vi "Periodic Tasks.vi"(8 "error in":errorcluster) -> ()   [LabVIEW 2018]
doc: "This VI runs in parallel to other tasks. It can contain as many user-defined periodic loops as you need. These can carry out PID or other sorts of timed response."
uses:
  <vilib>/Rock Robotics/WPI/ThirdParty/Phoenix-LabVIEW/Motor Controller/Controls/CTRE_Phoenix_MotorControl_ControlMode.ctl
  Robot Global Data.vi
  <vilib>/addons/control/pid/pid.llb/PID (DBL).vi
  <vilib>/Rock Robotics/WPI/ThirdParty/Phoenix-LabVIEW/Motor Controller/Get/CTRE_Phoenix_MotorController_GetVoltage.vi
  <vilib>/addons/control/pid/NI_PID_pid.lvlib
  <vilib>/Rock Robotics/SystemInterfaces/DIO/FPGA_DIOChannel.ctl
panel:
  in  "Front Center":i16=-81
  in  "Rear Center":i16=256
  out "Rear Encoder":i16=8
  out "Rear Encoder":dbl(graph)=8.0
  out "Front Encoder":i16=8
  out "Front Encoder":dbl(graph)=8.0
  in  "Initial Count":i32
  out "Count":dbl=-1091.0
  out "PID Output 2":dbl(graph)=0.5
  in  "Hue":cluster{dbl, dbl}(slide)={0.0, 5.05050505050505} scale=0.0..10.0
  in  "Saturation":cluster{dbl, dbl}(slide)={0.0, 5.05050505050505} scale=0.0..10.0
  in  "Value":cluster{dbl, dbl}(slide)={0.0, 5.05050505050505} scale=0.0..10.0
  in  "Count Offset":i32
  out "Counts":i32=1466
  out "Count State":dbl=-1091.0
  in  "Bucket PID":T1={"proportional gain (Kc)"=0.7, "integral time (Ti, min)"=0.0, "derivative time (Td, min)"=0.0}
  in  "PID Range":cluster{"output high":dbl, "output low":dbl}={"output high"=0.7, "output low"=-0.7} {"output low" format="%.2f"; "output high" format="%.2f"}
  out "PID Output":dbl(graph)=0.5
  out "PID Inputs":cluster{dbl, "Bucket Angle ":dbl}(graph)={-2182.0, "Bucket Angle "=0.0}
  out "Count Chart":cluster{dbl, "Value":i32}(graph)
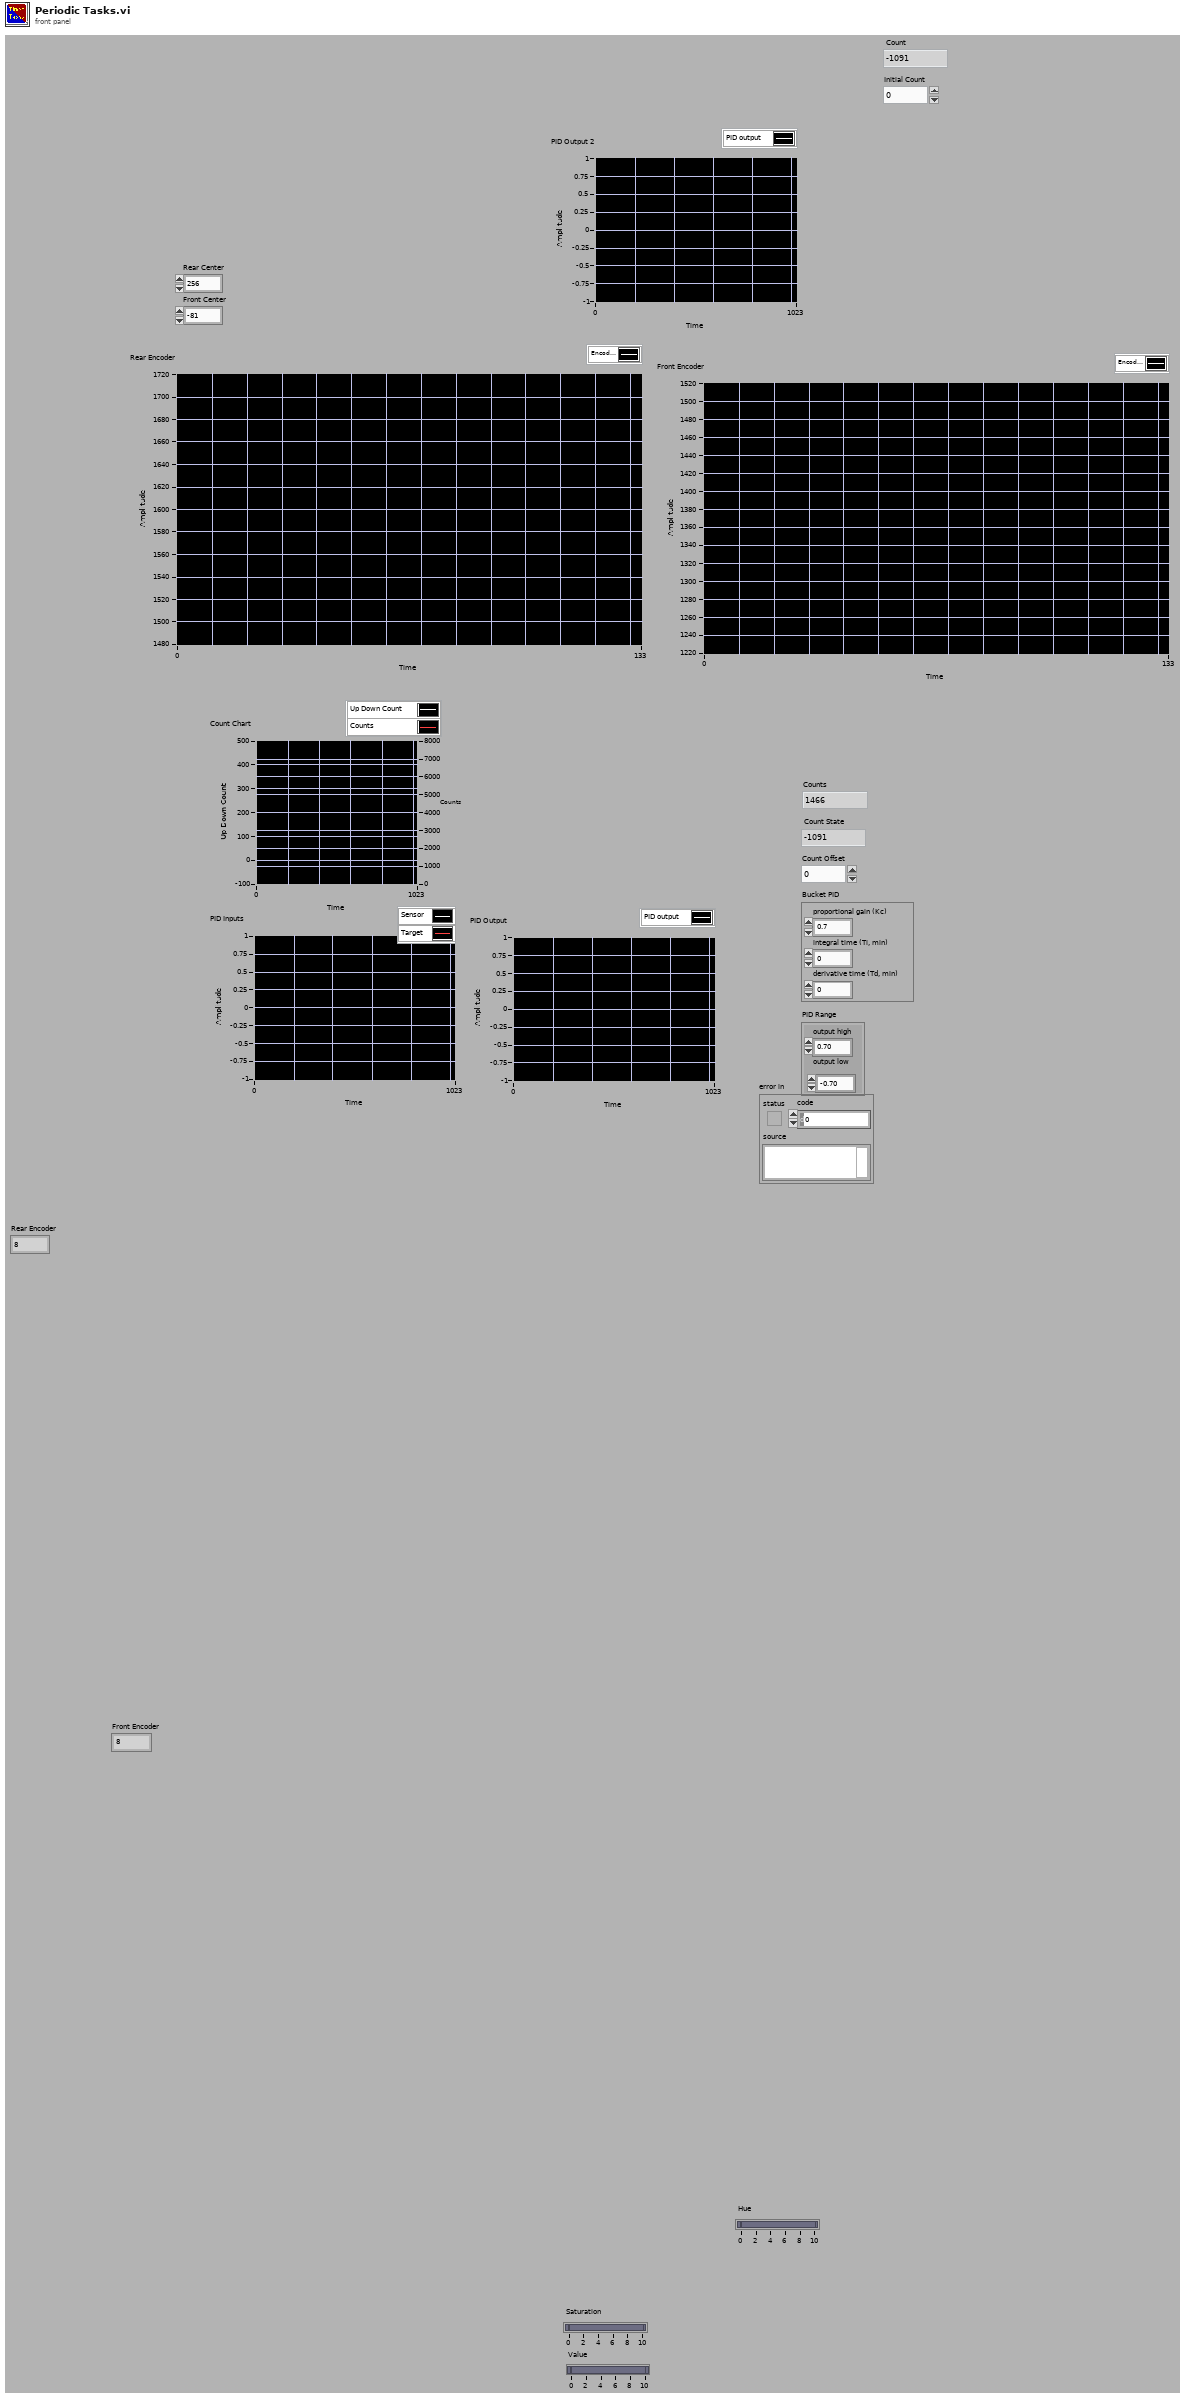
[diagram p1: front panel]
types:
  T1 = cluster{"proportional gain (Kc)":dbl, "integral time (Ti, min)":dbl, "derivative time (Td, min)":dbl}
  T2 = typedef "WPI_EncoderDevRef.ctl" = cluster{"DevStatus":errorcluster, "EncoderIndex":T3, "CounterIndex":T4, "DistancePerCount":dbl, "Decoding Type":T5}
  T3 = typedef "FPGA_EncoderIdx.ctl" = enum8{"Enc 0", "Enc 1", "Enc 2", "Enc 3", "Enc 4", "Enc 5", "Enc 6", "Enc 7", "Invalid"}
  T4 = typedef "FPGA_CounterCtrSystemIndex.ctl" = enum8{"Ctr 0", "Ctr 1", "Ctr 2", "Ctr 3", "Ctr 4", "Ctr 5", "Ctr 6", "Ctr 7", "Invalid"}
  T5 = typedef "WPI_EncoderType.ctl" = enum16{"1x", "2x", "4x"}
  T6 = typedef "WPI_MotorControlDeviceRef.ctl" = cluster{"DeviceStatus":errorcluster, "Type":T7, "PWM":cluster{"PWM Channel":T8, "DeadBand":T9}, "CAN":cluster{"Device Number":u8, "SetOutput VI Ref":variant, "GetOutput VI Ref":variant, "Enable VI Ref":variant, "Disable VI Ref":variant, "Data":variant}, "Invert":bool, "DIO PWM":cluster{"PWM \"Enable\" Channel":T8, "DIOChannel":T10, "PWM Rate":dbl}}
  T7 = typedef "WPI_MotorControlType.ctl" = enum16{"PWM", "CAN", "DIO PWM"}
  T8 = typedef "FPGA_DIOPWMChannel.ctl" = enum8{"PWM 0", "PWM 1", "PWM 2", "PWM 3", "PWM 4", "PWM 5", "PWM 6", "PWM 7", "PWM 8", "PWM 9", "PWM MXP 0", "PWM MXP 1", "PWM MXP 2", "PWM MXP 3", "PWM MXP 4", "PWM MXP 5", "PWM MXP 6", "PWM MXP 7", "PWM MXP 8", "PWM MXP 9", "Invalid"}
  T9 = typedef "WPI_PWMDeadband.ctl" = cluster{"Name":string, "maxPositivePwm":i32, "minPositivePwm":i32, "centerPwm":i32, "maxNegativePwm":i32, "minNegativePwm":i32, "angularRange":u16}
  T10 = typedef "FPGA_DIOChannel.ctl" = enum8{"DIO 0", "DIO 1", "DIO 2", "DIO 3", "DIO 4", "DIO 5", "DIO 6", "DIO 7", "DIO 8", "DIO 9", "DIO MXP 0", "DIO MXP 1", "DIO MXP 2", "DIO MXP 3", "DIO MXP 4", "DIO MXP 5", "DIO MXP 6", "DIO MXP 7", "DIO MXP 8", "DIO MXP 9", "DIO MXP 10", "DIO MXP 11", "DIO MXP 12", "DIO MXP 13", "DIO MXP 14", "DIO MXP 15", "SPI Port CS1", "SPI Port CS2", "SPI Port CS3", "SPI Port MISO", "SPI Port MOSI", "Invalid"}
  T11 = typedef "WPI_CounterDevRef.ctl" = cluster{"DevStatus":errorcluster, "CntIndex":T4}
  T12 = typedef "WPI_DigitalOutputDevRef.ctl" = cluster{"DIO Channel":T10, "DevStatus":errorcluster}
  T13 = typedef "CTRE_Phoenix_MotorControl_ControlMode.ctl" = u16
  T14 = typedef "WPI_SwitchDevRef.ctl" = cluster{"DevStatus":errorcluster, "DIO Channel":T10, "CntIndex":T4, "Normally Closed":bool}
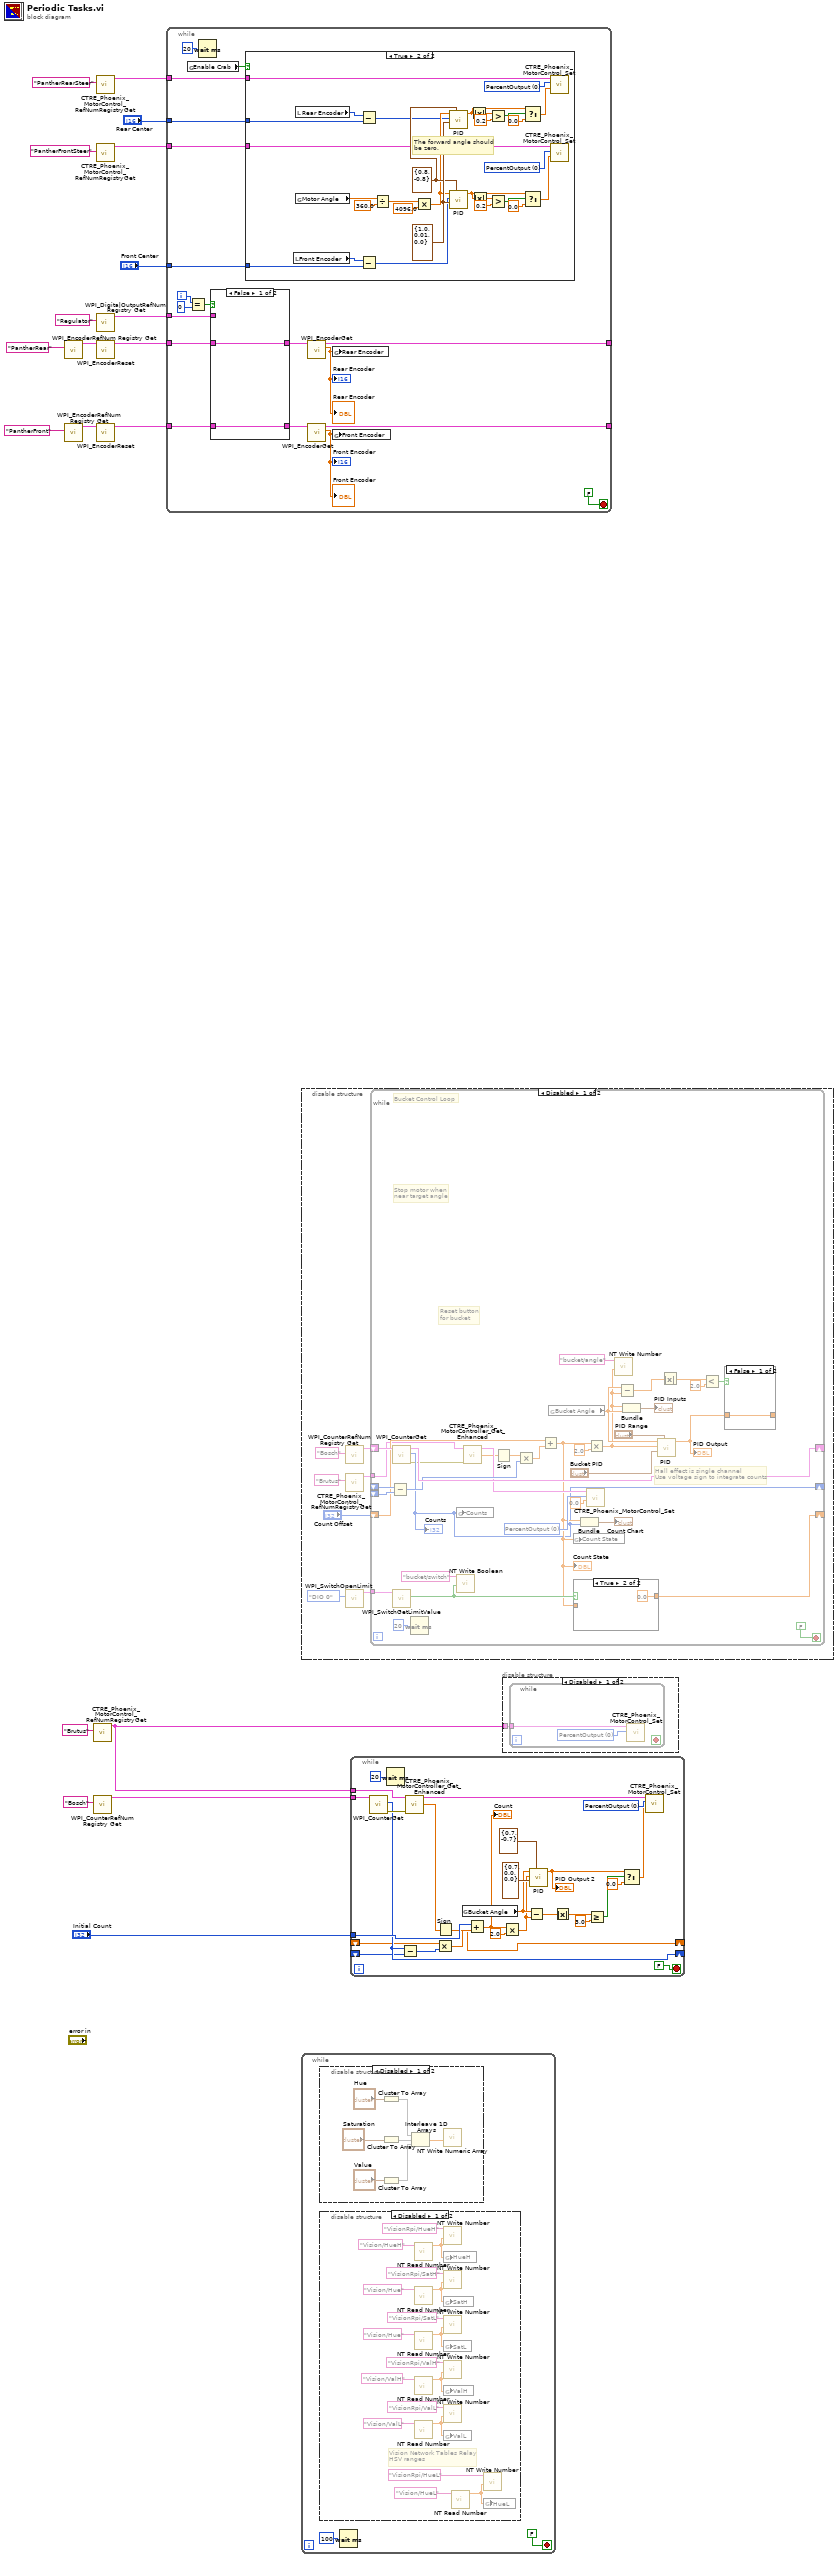
[diagram p0: block diagram]
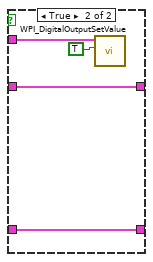
[diagram p2: hidden frame]
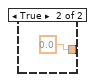
[diagram p5: hidden frame]
diagram:
  n1 = call <vilib>:"WPI_EncoderRefNum Registry Get.vi"("refnum name"="PantherRear") -> ("EncoderDevRef"=w10:T2)  [unwired: 9 in, 1 out]
  n2 = call <vilib>:"WPI_EncoderRefNum Registry Get.vi"("refnum name"="PantherFront") -> ("EncoderDevRef"=w12:T2)  [unwired: 9 in, 1 out]
  n3 = call <vilib>:"CTRE_Phoenix_MotorControl_RefNumRegistryGet.vi"("refnum name"="Brutus") -> ("PhoenixMotorControlDevRef"=w15:T6)  [unwired: 9 in, 1 out]
  n4 = call <vilib>:"WPI_CounterRefNum Registry Get.vi"("refnum name"="Bosch") -> ("CounterDevRef"=w16:T11)  [unwired: 9 in, 1 out]
  n5 = call <vilib>:"CTRE_Phoenix_MotorControl_RefNumRegistryGet.vi"("refnum name"="PantherRearSteer") -> ("PhoenixMotorControlDevRef"=w8:T6)  [unwired: 9 in, 1 out]
  n6 = call <vilib>:"CTRE_Phoenix_MotorControl_RefNumRegistryGet.vi"("refnum name"="PantherFrontSteer") -> ("PhoenixMotorControlDevRef"=w9:T6)  [unwired: 9 in, 1 out]
  n7 = call <vilib>:"WPI_DigitalOutputRefNum Registry Get.vi"("refnum name"="Regulator") -> ("DigitalOutputDevRef"=w5:T12)  [unwired: 9 in, 1 out]
  n8 = call <vilib>:"WPI_EncoderReset.vi"("EncoderDevRef"=w10) -> ("EncoderDevRef"=w3:T2)  [unwired: 9 in, 1 out]
  n9 = call <vilib>:"WPI_EncoderReset.vi"("EncoderDevRef"=w12) -> ("EncoderDevRef"=w4:T2)  [unwired: 9 in, 1 out]
  n10 = while {
    tunnel: w9 -> [w36]
    tunnel: w8 -> [w35]
    tunnel: w5 -> [w33]
    tunnel: w4 -> [w32]
    tunnel: w3 -> [w31]
    tunnel: [w24] -> _
    tunnel: [w23] -> _
    tunnel: "Rear Center" -> [w22]
    tunnel: "Front Center" -> [w21]
    i -> [w20]
    stop <- FALSE stop-if-true
    n11 = global read "Robot Global Data.vi" "Enable Crab"() -> (w34:bool)
    n12 = Equal?(x=w20, y=0) -> (x = y?=w29:bool)
    n13 = Wait (ms)(milliseconds to wait=u32 20) -> ()  [unwired: 1 out]
    n14 = case shown="False" w29 {
      tunnel: w33 -> [_ w44]
      tunnel: [w40 w42] -> w27
      tunnel: w32 -> [w40 w42]
      tunnel: [w39 w41] -> w25
      tunnel: w31 -> [w39 w41]
      frame False {
      }
      frame True {
        n15 = call <vilib>:"WPI_DigitalOutputSetValue.vi"("Value"=TRUE, "DigitalOutputDevRef"=w44) -> ()  [unwired: 8 in, 2 out]
      }
    }
    n16 = case shown="True" w34 {
      tunnel: w36 -> [_ w70]
      tunnel: w35 -> [_ w69]
      tunnel: w22 -> [_ w47]
      tunnel: w21 -> [_ w49]
      frame False {
      }
      frame True {
        w67 = T13 0 items=["PercentOutput"=0, "Position"=1, "Velocity"=2, "Current"=3, "Follower"=5, "MotionProfile"=6, "MotionMagic"=7, "MotionProfileArc"=10, "Disabled"=15] ("Control Mode")
        w68 = T13 0 items=["PercentOutput"=0, "Position"=1, "Velocity"=2, "Current"=3, "Follower"=5, "MotionProfile"=6, "MotionMagic"=7, "MotionProfileArc"=10, "Disabled"=15] ("Control Mode")
        w71 = cluster{"output high":dbl, "output low":dbl} {"output high"=0.8, "output low"=-0.8} ("output range")
        w73 = T1 {"proportional gain (Kc)"=1.0, "integral time (Ti, min)"=0.01, "derivative time (Td, min)"=0.0} ("PID gains")
        # "The forward angle should\nbe zero."
        n17 = local read "Front Encoder"() -> (w50:i16)
        n18 = local read "Rear Encoder"() -> (w72:i16)
        n19 = global read "Robot Global Data.vi" "Motor Angle"() -> (w66:dbl)
        n20 = Subtract(x=w72, y=w47) -> (x-y=w48:i16)
        n21 = Subtract(x=w50, y=w49) -> (x-y=w51:i16)
        n22 = Divide(x=w66, y=360.0) -> (x/y=w64:dbl)
        n23 = Multiply(x=w64, y=4096.0) -> (x*y=w62:dbl)
        n24 = call-poly <vilib>:"PID.vi"("output range"=w71, "PID gains"=w73, "process variable"=w48, "setpoint"=w62) -> ("output"=w52:dbl)  [unwired: 6 in, 1 out]
        n25 = call-poly <vilib>:"PID.vi"("output range"=w71, "PID gains"=w73, "process variable"=w51, "setpoint"=w62) -> ("output"=w61:dbl)  [unwired: 6 in, 1 out]
        n26 = Absolute Value(x=w52) -> (abs(x)=w46:dbl)
        n27 = Absolute Value(x=w61) -> (abs(x)=w45:dbl)
        n28 = Greater?(x=w46, y=0.2) -> (0:w56:bool)
        n29 = Greater?(x=w45, y=0.2) -> (0:w59:bool)
        n30 = Select(t=w52, s=w56, f=0.0) -> (s? t:f=w54:dbl)
        n31 = Select(t=w61, s=w59, f=0.0) -> (s? t:f=w53:dbl)
        n32 = call <vilib>:"CTRE_Phoenix_MotorControl_Set.vi"("Output"=w54, "Control Mode"=w68, "PhoenixMotorControlDevRef"=w69) -> ()  [unwired: 7 in, 2 out]
        n33 = call <vilib>:"CTRE_Phoenix_MotorControl_Set.vi"("Output"=w53, "Control Mode"=w67, "PhoenixMotorControlDevRef"=w70) -> ()  [unwired: 7 in, 2 out]
      }
    }
    n34 = call <vilib>:"WPI_EncoderGet.vi"("EncoderDevRef"=w25) -> ("Distance"=w26:dbl, "EncoderDevRef"=w23:T2)  [unwired: 5 in, 4 out]
    "Rear Encoder" <- w26
    "Rear Encoder" <- w26
    n35 = call <vilib>:"WPI_EncoderGet.vi"("EncoderDevRef"=w27) -> ("Distance"=w28:dbl, "EncoderDevRef"=w24:T2)  [unwired: 5 in, 4 out]
    "Front Encoder" <- w28
    "Front Encoder" <- w28
    n36 = global write "Robot Global Data.vi" "Rear Encoder"(w26) -> ()
    n37 = global write "Robot Global Data.vi" "Front Encoder"(w28) -> ()
  }
  n38 = disable-structure shown="Disabled" {
    frame Disabled {
      n39 = call <vilib>:"WPI_CounterRefNum Registry Get.vi"("refnum name"="Bosch") -> ("CounterDevRef"=w80:T11)  [unwired: 9 in, 1 out]
      n40 = call <vilib>:"CTRE_Phoenix_MotorControl_RefNumRegistryGet.vi"("refnum name"="Brutus") -> ("PhoenixMotorControlDevRef"=w78:T6)  [unwired: 9 in, 1 out]
      n41 = call <vilib>:"WPI_SwitchOpenLimit.vi"("DIO Channel"=FPGA_DIOChannel."DIO 0") -> ("SwitchDevRef"=w74:T14)  [unwired: 9 in, 1 out]
      n42 = while {
        shift-right: [w113] -> _
        shift-left: w80 -> [w115]
        tunnel: w78 -> [w101]
        shift-right: [w84] -> _
        shift-left: _ -> [w112]
        shift-left: _ -> [w111]
        shift-right: [w105] -> _
        shift-left: "Count Offset" -> [w110]
        tunnel: w74 -> [w90]
        stop <- FALSE stop-if-true
        w103 = T13 0 items=["PercentOutput"=0, "Position"=1, "Velocity"=2, "Current"=3, "Follower"=5, "MotionProfile"=6, "MotionMagic"=7, "MotionMagicArc"=8, "MotionProfileArc"=10, "Disabled"=15] ("Control Mode")
        # "Reset button\nfor bucket"
        # "Stop motor when\nnear target angle"
        # "Hall effect is single channel\nUse voltage sign to integrate counts"
        # "Bucket Control Loop"
        n43 = Subtract(x=w112, y=w111) -> (x-y=w109:i32)
        n44 = call <vilib>:"WPI_CounterGet.vi"("CounterDevRef in"=w115) -> ("error out"=w81:errorcluster, "Value"=w84:i32, "CounterDevRef out"=w113:T11)  [unwired: 5 in, 3 out]
        "Counts" <- w84
        n45 = call <vilib>:"WPI_SwitchGetLimitValue.vi"("SwitchDevRef"=w90) -> ("Switch Pressed"=w89:bool)  [unwired: 8 in, 2 out]
        n46 = Wait (ms)(milliseconds to wait=u32 20) -> ()  [unwired: 1 out]
        n47 = global write "Robot Global Data.vi" "Counts"(w84) -> ()
        n48 = call <vilib>:"NT Write Boolean.vi"("Boolean"=w89, "Name"="bucket/switch") -> ()  [unwired: 9 in, 1 out]
        n49 = call-poly <vilib>:"CTRE_Phoenix_MotorController_Get_Enhanced.vi"("PhoenixMotorControlDevRef"=w101, "error in"=w81) -> ("PhoenixMotorControlDevRef"=w100:T6, "Output Voltage"=w99:dbl)  [unwired: 9 in, 3 out]
        n50 = Sign(1:w99) -> (0:w98:dbl)
        n51 = Multiply(x=w98, y=w109) -> (x*y=w108:dbl)
        n52 = Add(x=w110, y=w108) -> (x+y=w85:dbl)
        "Count State" <- w85
        n53 = global read "Robot Global Data.vi" "Bucket Angle"() -> (w97:dbl)
        n54 = global write "Robot Global Data.vi" "Count State"(w85) -> ()
        n55 = case shown="True" w89 {
          tunnel: [w118 0.0] -> w105
          tunnel: w85 -> [w118 _]
          frame False {
          }
          frame True {
          }
        }
        n56 = Bundle(w85, "Value"=w84) -> (→"Count Chart":cluster{dbl, "Value":i32})  [unwired: 1 in]
        n57 = call <vilib>:"CTRE_Phoenix_MotorControl_Set.vi"("Output"=0.0, "Control Mode"=w103, "PhoenixMotorControlDevRef"=w100) -> ()  [unwired: 7 in, 2 out]
        n58 = Multiply(x=w85, y=2.0) -> (x*y=w87:dbl)
        n59 = call <vilib>:"NT Write Number.vi"("Numeric"=w87, "Name"="bucket/angle") -> ()  [unwired: 9 in, 1 out]
        n60 = Subtract(x=w97, y=w87) -> (x-y=w96:dbl)
        n61 = Bundle(w87, "Bucket Angle"=w97) -> (→"PID Inputs":cluster{dbl, "Bucket Angle":dbl})  [unwired: 1 in]
        n62 = call-poly <vilib>:"PID.vi"("output range"="PID Range", "PID gains"="Bucket PID", "process variable"=w87, "setpoint"=w97) -> ("output"=w92:dbl)  [unwired: 6 in, 1 out]
        "PID Output" <- w92
        n63 = Absolute Value(x=w96) -> (abs(x)=w94:dbl)
        n64 = Less?(x=w94, y=2.0) -> (x < y?=w95:bool)
        n65 = case shown="False" w95 {
          tunnel: w92 -> [w116 _]
          tunnel: [w116 0.0 ("output")] -> _
          frame False {
          }
          frame True {
          }
        }
      }
    }
    frame Enabled {
    }
  }
  n66 = while {
    stop <- FALSE stop-if-true
    n67 = disable-structure shown="Disabled" {
      frame Disabled {
        n68 = Cluster To Array(cluster="Hue") -> (array=w145:dbl[])
        n69 = Cluster To Array(cluster="Saturation") -> (array=w143:dbl[])
        n70 = Cluster To Array(cluster="Value") -> (array=w141:dbl[])
        n71 = Interleave 1D Arrays(w145, w143, w141) -> (w140:dbl[])
        n72 = call <vilib>:"NT Write Numeric Array.vi"("Numeric Array"=w140) -> ()  [unwired: 10 in, 1 out]
      }
      frame Enabled {
      }
    }
    n73 = disable-structure shown="Disabled" {
      frame Disabled {
        # "Vision Network Tables Relay\nHSV ranges"
        n74 = call <vilib>:"NT Read Number.vi"("Name"="Vision/HueH") -> ("Numeric"=w135:dbl)  [unwired: 9 in, 1 out]
        n75 = call <vilib>:"NT Read Number.vi"("Name"="Vision/Hue") -> ("Numeric"=w129:dbl)  [unwired: 9 in, 1 out]
        n76 = call <vilib>:"NT Read Number.vi"("Name"="Vision/Hue") -> ("Numeric"=w132:dbl)  [unwired: 9 in, 1 out]
        n77 = call <vilib>:"NT Read Number.vi"("Name"="Vision/ValH") -> ("Numeric"=w123:dbl)  [unwired: 9 in, 1 out]
        n78 = call <vilib>:"NT Read Number.vi"("Name"="Vision/ValL") -> ("Numeric"=w126:dbl)  [unwired: 9 in, 1 out]
        n79 = call <vilib>:"NT Write Number.vi"("Numeric"=w135, "Name"="VisionRpi/HueH") -> ()  [unwired: 9 in, 1 out]
        n80 = global write "Robot Global Data.vi" "HueH"(w135) -> ()
        n81 = call <vilib>:"NT Write Number.vi"("Numeric"=w129, "Name"="VisionRpi/SatH") -> ()  [unwired: 9 in, 1 out]
        n82 = global write "Robot Global Data.vi" "SatH"(w129) -> ()
        n83 = call <vilib>:"NT Write Number.vi"("Numeric"=w132, "Name"="VisionRpi/SatL") -> ()  [unwired: 9 in, 1 out]
        n84 = global write "Robot Global Data.vi" "SatL"(w132) -> ()
        n85 = call <vilib>:"NT Write Number.vi"("Numeric"=w123, "Name"="VisionRpi/ValH") -> ()  [unwired: 9 in, 1 out]
        n86 = global write "Robot Global Data.vi" "ValH"(w123) -> ()
        n87 = call <vilib>:"NT Write Number.vi"("Numeric"=w126, "Name"="VisionRpi/ValL") -> ()  [unwired: 9 in, 1 out]
        n88 = global write "Robot Global Data.vi" "ValL"(w126) -> ()
        n89 = call <vilib>:"NT Read Number.vi"("Name"="Vision/HueL") -> ("Numeric"=w138:dbl)  [unwired: 9 in, 1 out]
        n90 = call <vilib>:"NT Write Number.vi"("Numeric"=w138, "Name"="VisionRpi/HueL") -> ()  [unwired: 9 in, 1 out]
        n91 = global write "Robot Global Data.vi" "HueL"(w138) -> ()
      }
      frame Enabled {
      }
    }
    n92 = Wait (ms)(milliseconds to wait=u32 100) -> ()  [unwired: 1 out]
  }
  n93 = while {
    tunnel: w15 -> [w166]
    tunnel: w16 -> [w156]
    shift-right: [w155] -> _
    shift-left: _ -> [w154]
    shift-right: [w153] -> _
    shift-left: _ -> [w152]
    tunnel: "Initial Count" -> [w173]
    stop <- FALSE stop-if-true
    w167 = T13 0 items=["PercentOutput"=0, "Position"=1, "Velocity"=2, "Current"=3, "Follower"=5, "MotionProfile"=6, "MotionMagic"=7, "MotionMagicArc"=8, "MotionProfileArc"=10, "Disabled"=15] ("Control Mode")
    n94 = call <vilib>:"WPI_CounterGet.vi"("CounterDevRef in"=w156) -> ("error out"=w157:errorcluster, "Value"=w155:i32)  [unwired: 5 in, 4 out]
    n95 = Wait (ms)(milliseconds to wait=u32 20) -> ()  [unwired: 1 out]
    n96 = Subtract(x=w155, y=w154) -> (x-y=w172:i32)
    n97 = call-poly <vilib>:"CTRE_Phoenix_MotorController_Get_Enhanced.vi"("PhoenixMotorControlDevRef"=w166, "error in"=w157) -> ("PhoenixMotorControlDevRef"=w165:T6, "Output Voltage"=w164:dbl)  [unwired: 9 in, 3 out]
    n98 = Multiply(x=w152, y=w172) -> (x*y=w171:dbl)
    n99 = Sign(1:w164) -> (0:w153:dbl)
    n100 = global read "Robot Global Data.vi" "Bucket Angle"() -> (w163:dbl)
    n101 = Add(x=w173, y=w171) -> (x+y=w158:dbl)
    "Count" <- w158
    n102 = Multiply(x=w158, y=2.0) -> (x*y=w159:dbl)
    n103 = Subtract(x=w163, y=w159) -> (x-y=w162:dbl)
    n104 = call-poly <vilib>:"PID.vi"("output range"=cluster{"output high":dbl, "output low":dbl} {"output high"=0.7, "output low"=-0.7} ("PID Range 2"), "PID gains"=T1 {"proportional gain (Kc)"=0.7, "integral time (Ti, min)"=0.0, "derivative time (Td, min)"=0.0} ("Bucket PID 2"), "process variable"=w159, "setpoint"=w163) -> ("output"=w150:dbl)  [unwired: 6 in, 1 out]
    "PID Output 2" <- w150
    n105 = Absolute Value(x=w162) -> (abs(x)=w161:dbl)
    n106 = Greater Or Equal?(x=w161, y=3.0) -> (x >= y?=w151:bool)
    n107 = Select(t=w150, s=w151, f=0.0) -> (s? t:f=w148:dbl)
    n108 = call <vilib>:"CTRE_Phoenix_MotorControl_Set.vi"("Output"=w148, "Control Mode"=w167, "PhoenixMotorControlDevRef"=w165) -> ()  [unwired: 7 in, 2 out]
  }
  n109 = disable-structure shown="Disabled" {
    disable-tunnel: w15 -> [w175 _]
    frame Disabled {
      n110 = while {
        tunnel: w175 -> [w176]
        stop <- _ stop-if-true
        w177 = T13 0 items=["PercentOutput"=0, "Position"=1, "Velocity"=2, "Current"=3, "Follower"=5, "MotionProfile"=6, "MotionMagic"=7, "MotionMagicArc"=8, "MotionProfileArc"=10, "Disabled"=15] ("Control Mode")
        n111 = call <vilib>:"CTRE_Phoenix_MotorControl_Set.vi"("Control Mode"=w177, "PhoenixMotorControlDevRef"=w176) -> ()  [unwired: 8 in, 2 out]
      }
    }
    frame Enabled {
    }
  }
